vi "ingest.video-without_manifest_timestamp.vi"(6 "Properties and Labels":T1, 7 "Starting Timestamp":timestamp format="%<%x %.3X>T", 8 "error in":errorcluster, 9 "Title and Description":cluster{"Title":string, "Description":string}, 10 "S3 Path":string, 11 "Nominal Client in":refnum<class "Nominal Client.lvclass">) -> (0 "error out":errorcluster, 1 "Response":T2, 2 "Video RID":string, 3 "Nominal Client out":refnum<class "Nominal Client.lvclass">, 4 "Response":string)   [LabVIEW 2020, in "Nominal Client.lvclass"]
doc: "Ingests video data from a S3 Nominal upload bucket."
uses:
  Nominal Client.lvclass
  7ff8c0e1-378e-498f-a1ee-cc23b49038c3.vi
  328a2a72-b35c-448c-8cc8-7fb2a3abc54b.vi
  03f47964-3351-4de7-ad21-2429850d9a88.vi
  4b965f09-dc68-4d5e-a5c1-32d476accfd4.vi
  <vilib>/LabVIEW Open Source Project/Epoch Date & Time/epoch.UNIX/Epoch.UNIX.lvclass
  C:/Program Files/National Instruments/LabVIEW 2020/vi.lib/LabVIEW Open Source Project/Epoch Date & Time/epoch/Epoch.lvclass
  <vilib>/LabVIEW Open Source Project/Epoch Date & Time/Get Epoch Time.vi
  <vilib>/JDP Science/JSONtext/Variant to JSON Text.vi
  <vilib>/JDP Science/JSONtext/Array of Variants to JSON Object.vi
  <vilib>/JDP Science/JSONtext/Set Item.vi
  <vilib>/JDP Science/JSONtext/JSON text to Variant.vi
  <vilib>/JDP Science/JSONtext/LVClass Serializer/JSONtext LVClass Serializer.lvclass
  Nominal Client.lvclass/Nominal Client.ctl
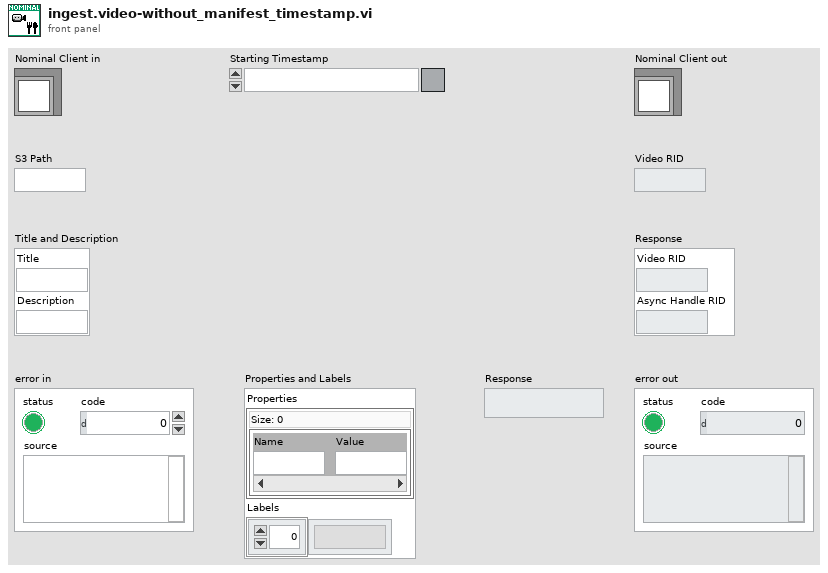
[diagram p1: front panel]
types:
  T1 = cluster{"Properties":map{string, string}, "Labels":string[]}
  T2 = cluster{"Video RID":string, "Async Handle RID":string}
  T3 = cluster{"type":string, "s3":cluster{"path":string}}[]
  T4 = cluster{"type":string, "noManifest":cluster{"startingTimestamp":cluster{"secondsSinceEpoch":i32, "offsetNanoseconds":i32}}}
  T5 = cluster{"videoRid":string, "asyncHandle":cluster{"rid":string}}
  T6 = cluster{"type":string, "s3":cluster{"path":string}}
  T7 = cluster{"sources":cluster{"type":string, "s3":cluster{"path":string}}[], "properties":string, "labels":string[], "timestamps":cluster{"type":string, "noManifest":cluster{"startingTimestamp":cluster{"secondsSinceEpoch":i32, "offsetNanoseconds":i32}}}, "title":string, "description":string}
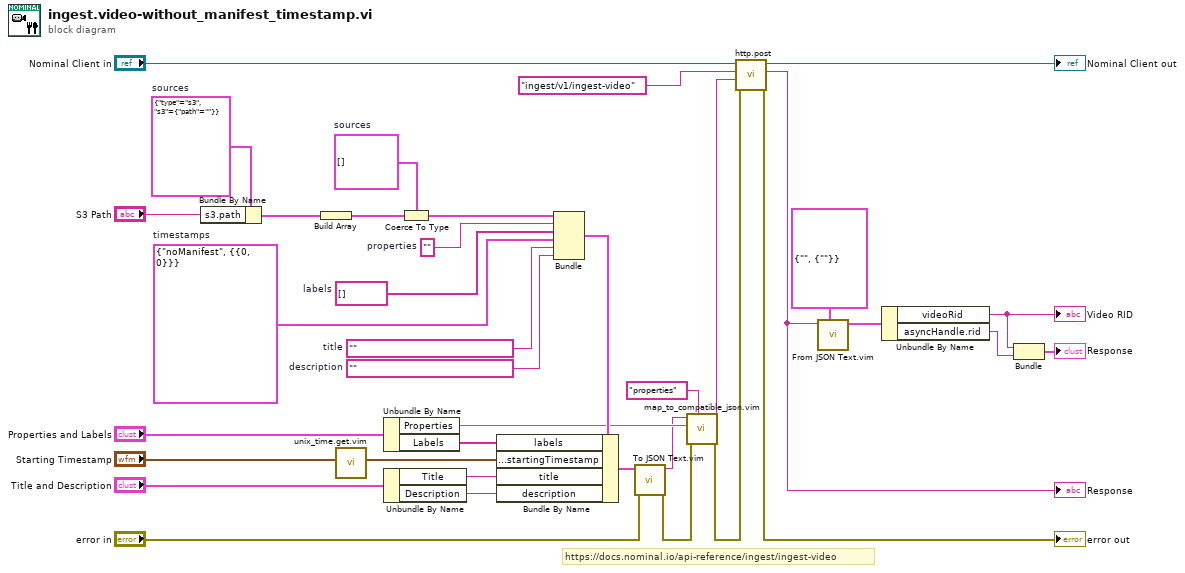
[diagram p0: block diagram]
diagram:
  w3 = T3 []  # sources
  w14 = ""  # properties
  w24 = ""  # description
  w25 = ""  # title
  w26 = T4 {"type"="noManifest", "noManifest"={"startingTimestamp"={"secondsSinceEpoch"=0, "offsetNanoseconds"=0}}}  # timestamps
  w27 = string[] []  # labels
  w8 = T6 {"type"="s3", "s3"={"path"=""}}  # sources
  # "https://docs.nominal.io/api-reference/ingest/ingest-video"
  n1 = Bundle By Name(cluster=w8, "s3.path"="S3 Path") -> (w6:T6)
  n2 = Build Array(w6) -> (w5:T3)
  n3 = call "unix_time.get.vim"("Time Stamp (empty: now) [single or array]"="Starting Timestamp") -> ("UNIX Timestamp"=w1:cluster{"Seconds":i64, "Nanoseconds":i64})  [unwired: 10 in]
  n4 = Unbundle By Name("Properties and Labels") -> ("Properties"=w15:map{string, string}, "Labels"=w19:string[])
  n5 = Unbundle By Name("Title and Description") -> ("Title"=w18:string, "Description"=w17:string)
  n6 = Coerce To Type(0:w5, 1:w3) -> (2:w4:T3)
  n7 = Bundle("sources"=w4, "properties"=w14, "labels"=w27, "timestamps"=w26, "title"=w25, "description"=w24) -> (w23:T7)  [unwired: 1 in]
  n8 = Bundle By Name(cluster=w23, "labels"=w19, "timestamps.noManifest.startingTimestamp"=w1, "title"=w18, "description"=w17) -> (w20:T7)
  n9 = call "To JSON Text.vim"("error in (no error)"="error in", "Anything"=w20) -> ("error out"=w10:errorcluster, "<JSON>"=w13:string)  [unwired: 8 in]
  n10 = call "map_to_compatible_json.vim"("JSON Path"="properties" ("Data Name"), "error in"=w10, "Map"=w15, "JSON in"=w13) -> ("error out"=w9:errorcluster, "JSON out"=w12:string)  [unwired: 6 in]
  n11 = call "http.post.vi"("error in"=w9, "Request body"=w12, "Path"="ingest/v1/ingest-video", "Nominal Client in"="Nominal Client in") -> ("error out"=→"error out":errorcluster, "Response"=w32:string, "Nominal Client out"=→"Nominal Client out":refnum<class "Nominal Client.lvclass">)  [unwired: 4 in, 1 out]
  "Response" <- w32
  n12 = call "From JSON Text.vim"("Data Type and Default Value"=T5 {"videoRid"="", "asyncHandle"={"rid"=""}} ("Information"), "JSON"=w32) -> ("Data out"=w31:T5)  [unwired: 8 in, 1 out]
  n13 = Unbundle By Name(w31) -> ("videoRid"=w30:string, "asyncHandle.rid"=w29:string)
  "Video RID" <- w30
  n14 = Bundle("videoRid"=w30, "rid"=w29) -> (→"Response":cluster{"videoRid":string, "rid":string})  [unwired: 1 in]
